vi "Get VI name.vi"(11 "VI in":refnum<vi>) -> (1 "Full Vi Name":string, 2 "Plain Name":string, 3 "VI out":refnum<vi>)   [LabVIEW 2019, in "Panther Dashboard.lvlib"]
uses:
  Panther Dashboard.lvlib
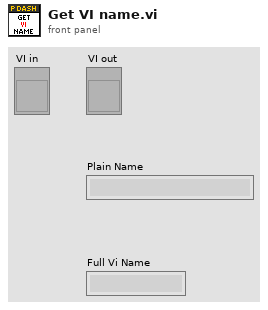
[diagram p1: front panel]
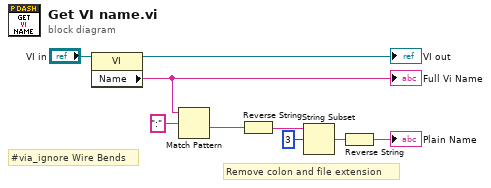
[diagram p0: block diagram]
diagram:
  # "#via_ignore Wire Bends"
  # "Remove colon and file extension"
  n1 = property class="VI"(reference="VI in") -> (reference out=→"VI out":refnum<vi>, "Name"=w1:string)  [unwired: 1 in, 1 out]
  "Full Vi Name" <- w1
  n2 = Match Pattern(string=w1, regular expression=":") -> (after substring=w7:string)  [unwired: 1 in, 3 out]
  n3 = Reverse String(1:w7) -> (0:w4:string)
  n4 = String Subset(string=w4, offset (0)=3) -> (substring=w3:string)  [unwired: 1 in]
  n5 = Reverse String(1:w3) -> (0:→"Plain Name":string)
